vi "ttm_lightIndicator_poller.vi"() -> ()   [LabVIEW 2010]
panel:
  out "Cyclic":bool
  out "Ramp":bool
  out "Logging is on":bool
  out "Measurement is going on":bool
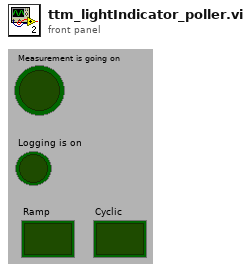
[diagram p1: front panel]
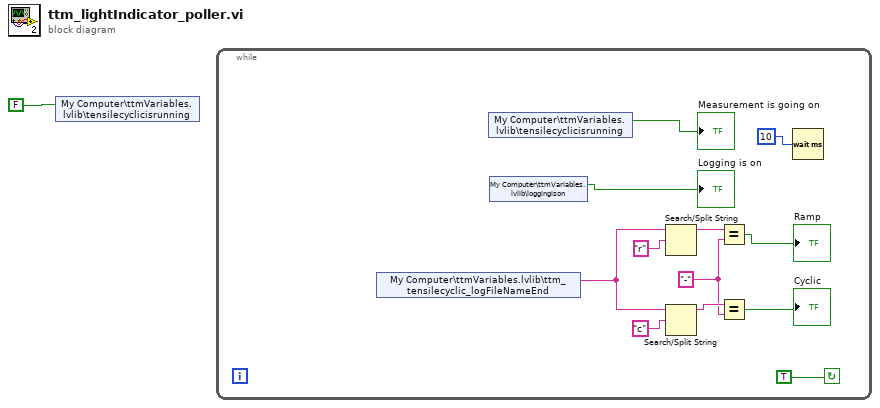
[diagram p0: block diagram]
diagram:
  n1 = shared-variable "My Computer\\ttmVariables.lvlib\\tensilecyclicisrunning"(FALSE ("tensilecyclicisrunning")) -> ()  [unwired: 1 in, 1 out]
  n2 = while {
    stop <- TRUE continue-if-true
    w8 = "-"
    n3 = shared-variable "My Computer\\ttmVariables.lvlib\\ttm_tensilecyclic_logFileNameEnd"() -> (w7:string)  [unwired: 1 in, 1 out]
    n4 = shared-variable "My Computer\\ttmVariables.lvlib\\tensilecyclicisrunning"() -> (→"Measurement is going on":bool)  [unwired: 1 in, 1 out]
    n5 = shared-variable "My Computer\\ttmVariables.lvlib\\loggingison"() -> (→"Logging is on":bool)  [unwired: 1 in, 1 out]
    n6 = Search/Split String(string=w7, search string/char (-)="r") -> (substring before match=w9:string)  [unwired: 1 in, 2 out]
    n7 = Search/Split String(string=w7, search string/char (-)="c") -> (substring before match=w10:string)  [unwired: 1 in, 2 out]
    n8 = Equal?(x=w9, y=w8) -> (x = y?=→"Ramp":bool)
    n9 = Equal?(x=w10, y=w8) -> (x = y?=→"Cyclic":bool)
    n10 = Wait (ms)(milliseconds to wait=u32 10) -> ()  [unwired: 1 out]
  }
